vi "Write Bank Type.vi"(9 "Bank Type":T1, 11 "Bank in":refnum<class "Bank.lvclass">) -> (3 "Bank out":refnum<class "Bank.lvclass">)   [LabVIEW 2019, in "Bank.lvclass"]
uses:
  Bank.lvclass
  Bank Type.ctl
  Bank.lvclass/Bank.ctl
  <vilib>/rvi/eio/common/nirviEmuTemplateMethod_errors.vi
  <vilib>/eio/EIOMethodNode/EIOMethodNode.xnode
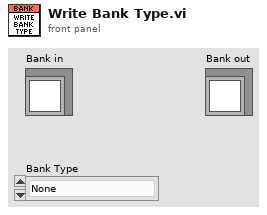
[diagram p1: front panel]
types:
  T1 = typedef "Bank.lvclass/Bank Type.ctl" = enum16{"None", "Discrete Acquisition", "Discrete Generation", "PWM Acquisition", "PWM Generation"}
  T2 = typedef "Bank.lvclass/DIO Resources.ctl" = cluster{"DIO 0":refnum<k21>, "DIO 1":refnum<k21>, "DIO 2":refnum<k21>, "DIO 3":refnum<k21>, "DIO 4":refnum<k21>, "DIO 5":refnum<k21>, "DIO 6":refnum<k21>, "DIO 7":refnum<k21>}
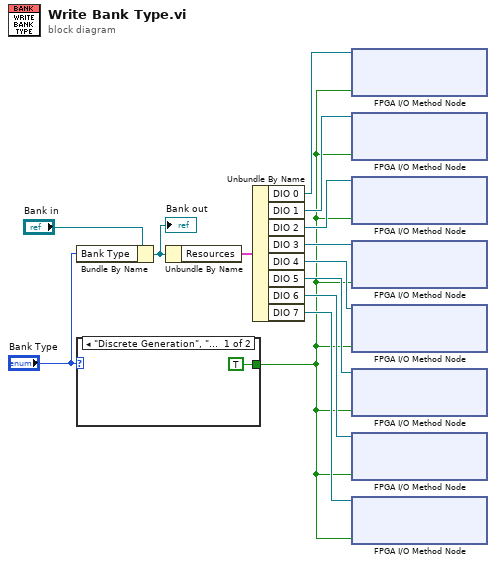
[diagram p0: block diagram]
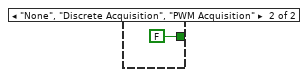
[diagram p2: hidden frame]
diagram:
  n1 = Bundle By Name(cluster="Bank in", "Bank Type"="Bank Type") -> (w12:refnum<class "Bank.lvclass">)
  "Bank out" <- w12
  n2 = case shown="\"Discrete Generation\", \"PWM Generation\"" "Bank Type" {
    tunnel: [TRUE ("Enable") FALSE ("Enable")] -> w1
    frame "Discrete Generation", "PWM Generation" {
    }
    frame "None", "Discrete Acquisition", "PWM Acquisition" {
    }
  }
  n3 = Unbundle By Name(w12) -> ("Resources"=w10:T2)
  n4 = Unbundle By Name(w10) -> ("DIO 0"=w9:refnum<k21>, "DIO 1"=w8:refnum<k21>, "DIO 2"=w7:refnum<k21>, "DIO 3"=w6:refnum<k21>, "DIO 4"=w5:refnum<k21>, "DIO 5"=w4:refnum<k21>, "DIO 6"=w3:refnum<k21>, "DIO 7"=w2:refnum<k21>)
  n5 = xnode "FPGA I/O Method Node"("FPGA I/O In"=w9, "Enable"=w1) -> ()  [unwired: 1 out]
  n6 = xnode "FPGA I/O Method Node"("FPGA I/O In"=w8, "Enable"=w1) -> ()  [unwired: 1 out]
  n7 = xnode "FPGA I/O Method Node"("FPGA I/O In"=w7, "Enable"=w1) -> ()  [unwired: 1 out]
  n8 = xnode "FPGA I/O Method Node"("FPGA I/O In"=w6, "Enable"=w1) -> ()  [unwired: 1 out]
  n9 = xnode "FPGA I/O Method Node"("FPGA I/O In"=w5, "Enable"=w1) -> ()  [unwired: 1 out]
  n10 = xnode "FPGA I/O Method Node"("FPGA I/O In"=w4, "Enable"=w1) -> ()  [unwired: 1 out]
  n11 = xnode "FPGA I/O Method Node"("FPGA I/O In"=w3, "Enable"=w1) -> ()  [unwired: 1 out]
  n12 = xnode "FPGA I/O Method Node"("FPGA I/O In"=w2, "Enable"=w1) -> ()  [unwired: 1 out]
